vi "initialise.vi"(8 "error in (no error)":errorcluster, 11 "WriteSignalsDAQmxPlugin in":refnum<class "SignalWriterMM140725DAQmx.lvclass">) -> (0 "error out":errorcluster, 3 "WriteSignalsDAQmxPlugin out":refnum<class "SignalWriterMM140725DAQmx.lvclass">)   [LabVIEW 2010, in "SignalWriterMM140725DAQmx.lvclass"]
uses:
  SignalWriterMM140725DAQmx.lvclass
  GenericSignalWriter/GenericSignalWriter/GenericSignalWriter.lvclass
  common/enumerations/functional_global_action_enum.ctl
  Program Files (x86)/National Instruments/LabVIEW 2010/resource/objmgr/daqmx.rc
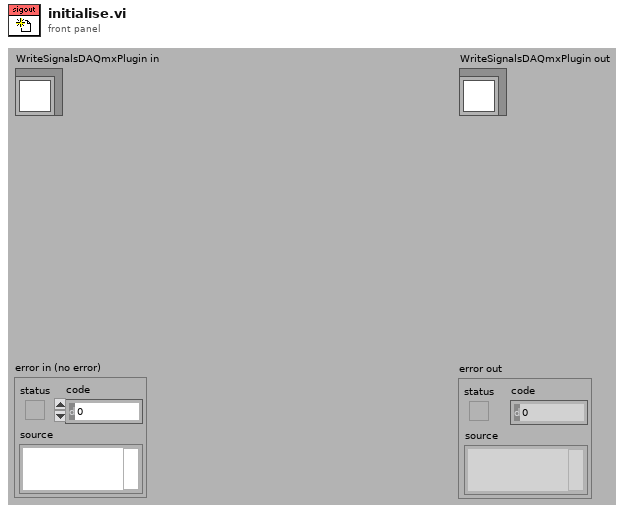
[diagram p1: front panel]
types:
  T1 = typedef "functional_global_action_enum.ctl" = enum16{"get", "set", "reset"}
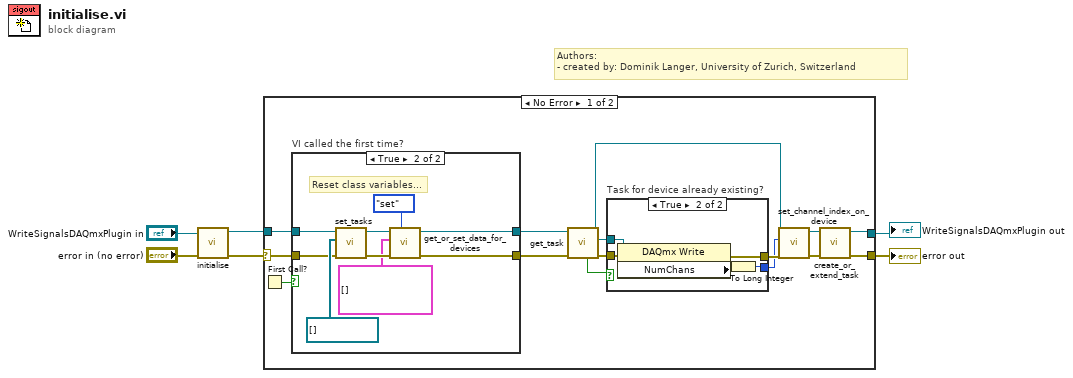
[diagram p0: block diagram]
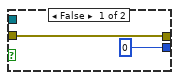
[diagram p2: hidden frame]
diagram:
  # "Authors: \n- created by: Dominik Langer, University of Zurich, Switzerland"
  n1 = call-parent "initialise.vi"("error in (no error)"="error in (no error)", "GenericPlugin in"="WriteSignalsDAQmxPlugin in") -> ("error out"=w4:errorcluster, "GenericPlugin out"=w2:refnum<class "SignalWriterMM140725DAQmx.lvclass">)  [unwired: 2 in, 6 out]
  n2 = case shown="No Error" w4 {
    selector: w4 -> [w21 w41]
    tunnel: [w10 w41] -> w3
    tunnel: [w9 w40] -> w1
    tunnel: w2 -> [w19 w40]
    frame No Error {
      n3 = First Call?() -> (First Call?: T/F=w20:bool)
      n4 = case "VI called the first time?" shown="True" w20 {
        tunnel: w21 -> [w30 w38]
        tunnel: [w30 w31] -> w8
        tunnel: w19 -> [w29 w37]
        tunnel: [w29 w34] -> w7
        frame False {
        }
        frame True {
          # "Reset class variables..."
          n5 = call-dynamic "set_tasks.vi"("error in (no error)"=w38, "output tasks"=refnum<k21>[] [] ("analog output tasks"), "DAQmxWriteSignals in"=w37) -> ("error out"=w36:errorcluster, "DAQmxWriteSignals out"=w35:refnum<class "SignalWriterMM140725DAQmx.lvclass">)  [unwired: 1 in, 6 out]
          n6 = call-dynamic "get_or_set_data_for_devices.vi"("action"=functional_global_action_enum."set", "error in (no error)"=w36, "data for devices in"=cluster{"data for channels":dbl[][]}[] [] ("data for devices"), "DAQmxWriteSignals in"=w35) -> ("error out"=w31:errorcluster, "DAQmxWriteSignals out"=w34:refnum<class "SignalWriterMM140725DAQmx.lvclass">)  [unwired: 6 out]
        }
      }
      n7 = call-dynamic "get_task.vi"("error in (no error)"=w8, "DAQmxWriteSignals in"=w7) -> ("error out"=w18:errorcluster, "writer task"=w17:refnum<k21>, "DAQmxWriteSignals out"=w13:refnum<class "SignalWriterMM140725DAQmx.lvclass">, "found?"=w16:bool)  [unwired: 6 out]
      n8 = case "Task for device already existing?" shown="True" w16 {
        tunnel: w18 -> [w22 w26]
        tunnel: [w22 w28] -> w15
        tunnel: [0 ("NumChans") w25] -> w14
        tunnel: w17 -> [_ w27]
        frame False {
        }
        frame True {
          n9 = property class="DAQmx Write"(reference=w27, error in=w26) -> (error out=w28:errorcluster, "NumChans"=w24:u32)  [unwired: 1 out]
          n10 = To Long Integer(number=w24) -> (32bit integer=w25:i32)
        }
      }
      n11 = call-dynamic "set_channel_index_on_device.vi"("error in (no error)"=w15, "channel index on device"=w14, "DAQmxWriteSignals.lvclass in"=w13) -> ("error out"=w12:errorcluster, "DAQmxWriteSignals.lvclass out"=w11:refnum<class "SignalWriterMM140725DAQmx.lvclass">)  [unwired: 7 out]
      n12 = call-dynamic "create_or_extend_task.vi"("error in (no error)"=w12, "DAQmxWriteSignals in"=w11) -> ("error out"=w10:errorcluster, "DAQmxWriteSignals out"=w9:refnum<class "SignalWriterMM140725DAQmx.lvclass">)  [unwired: 8 out]
    }
    frame Error {
    }
  }
  "error out" <- w3
  "WriteSignalsDAQmxPlugin out" <- w1
